vi "Control - Generic - Lambda Command Host.vi"() -> ()   [LabVIEW 2015, in "ECS-Host.lvlib"]
uses:
  ECS-Host.lvlib
  <vilib>/addons/Software Calibration Management/XControls/TBL2D.xctl
panel:
  in  "WvfrmAmp":sgl caption="[]"
  in  "WvfrmFreq":sgl caption="[]"
  in  "OscillationMode":enum32{"a", "b", "c", "d"}(ring)
  out "Lambda_Des":sgl caption="[]"
  in  "Lambda_Man":sgl caption="[]"
  in  "Lambda_ManE":bool
  out "Lambda_TblOut":sgl caption="[]"
  in  "Lambda_Tbl":cluster{"X":sgl[], "Y":sgl[], "Z":sgl[][]}(xcontrol)
  # "Lambda Calibration"
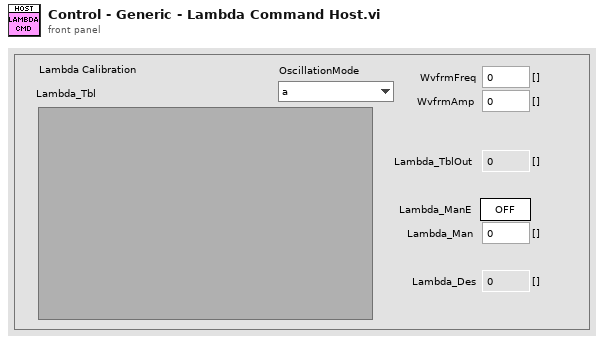
[diagram p1: front panel]
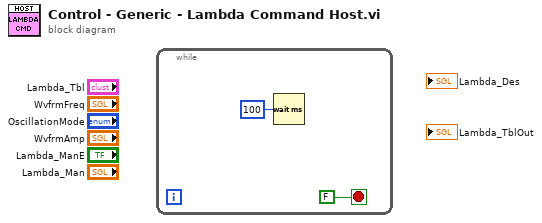
[diagram p0: block diagram]
diagram:
  n1 = while {
    stop <- FALSE stop-if-true
    n2 = Wait (ms)(milliseconds to wait=u32 100) -> ()  [unwired: 1 out]
  }
